vi "CPP_Aeroprobe_TimeSeries-AeroFlow.vi"() -> (5 "Plug in titles":string[](array[string]), 7 "Plug in values":string[](array[string]))   [LabVIEW 2021]
uses:
  Globals/Meas_global.vi
panel:
  in  "Downsampler":i32=10
  in  "Graphs":bool=TRUE
  out "AvgReduction (ms)":dbl
  out "reduction ms":u32
  in  "Correction File Path":path=path "M:/Preferences/Rig_Setups/All_Rigs/TubingCompensation/5HPTubingCorrection12066.xls"
  in  "Apply Phase Correction?":bool=TRUE
  out "DataArray":dbl[](array[numeric])
  out "Zeroes":dbl[](array[numeric])
  # "!! 5-hole 1-5 must be connected to Channels 1-5 !!"
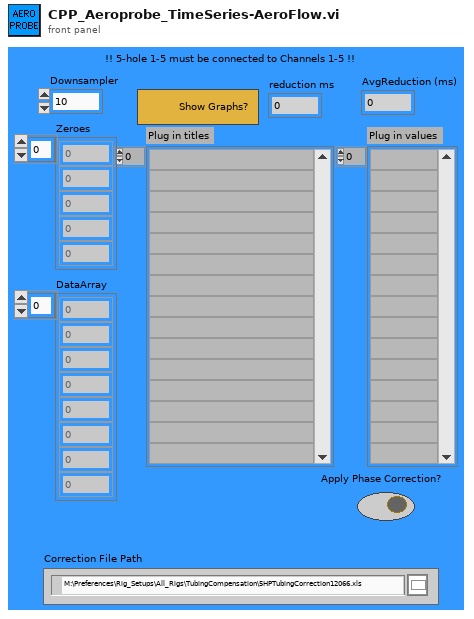
[diagram p1: front panel]
types:
  T1 = typedef "Analysis_info_cluster.ctl" = cluster{"Colour":u32, "Inst type":T2, "Inst name":string, "Symbol":string, "Code name":string, "Extra Info":string, "Inst Array":T3, "Extra Titles":string[], "Extra Values":string[], "U":dbl, "u^2":dbl, "u^3":dbl, "u^4":dbl, "Skew_u":dbl, "Kurt_u":dbl, "Sd Error in Mean":dbl, "% u'/U":dbl, "X":dbl, "Y":dbl, "Z":dbl, "Timescale integral to 25%":dbl, "Sd Error in Variance":dbl, "Calib File":path, "Calib Constants":dbl[], "Output Position":bool, "Full Stats":bool, "Av Sampling Rate":dbl, "Av No of Samples":dbl, "Total Meas Time (s)":dbl, "ADAM Ch Name":string}
  T2 = typedef "Inst_type.ctl" = enum16{"Propeller anemometer", "Raw voltage", "Pressure Transducer", "Pitot-static tube", "Preston tube", "Hot wire", "Cross wire 1", "Cross wire 2", "Generic Linear", "Generic Polynomial", "Generic BackPoly", "Fast FID", "Thermocouple", "Cold wire", "Pulsed Wire", "LDA Vel", "LDA Tran time", "LDA Arr time"}
  T3 = typedef "Instrument_Array.ctl" = enum16{"PWA", "LDA", "Analogue"}
  T4 = cluster{"Analysis Info cluster[0]":T1, "Analysis Info cluster[1]":T1, "Analysis Info cluster[2]":T1, "Analysis Info cluster[3]":T1, "Analysis Info cluster[4]":T1, "Analysis Info cluster[5]":T1, "Analysis Info cluster[6]":T1}
  T5 = typedef "Time_Trace_Cluster.ctl" = cluster{"Weighting":dbl[], "Time (s)":dbl[], "Voltage":dbl[], "Eng Values":dbl[]}
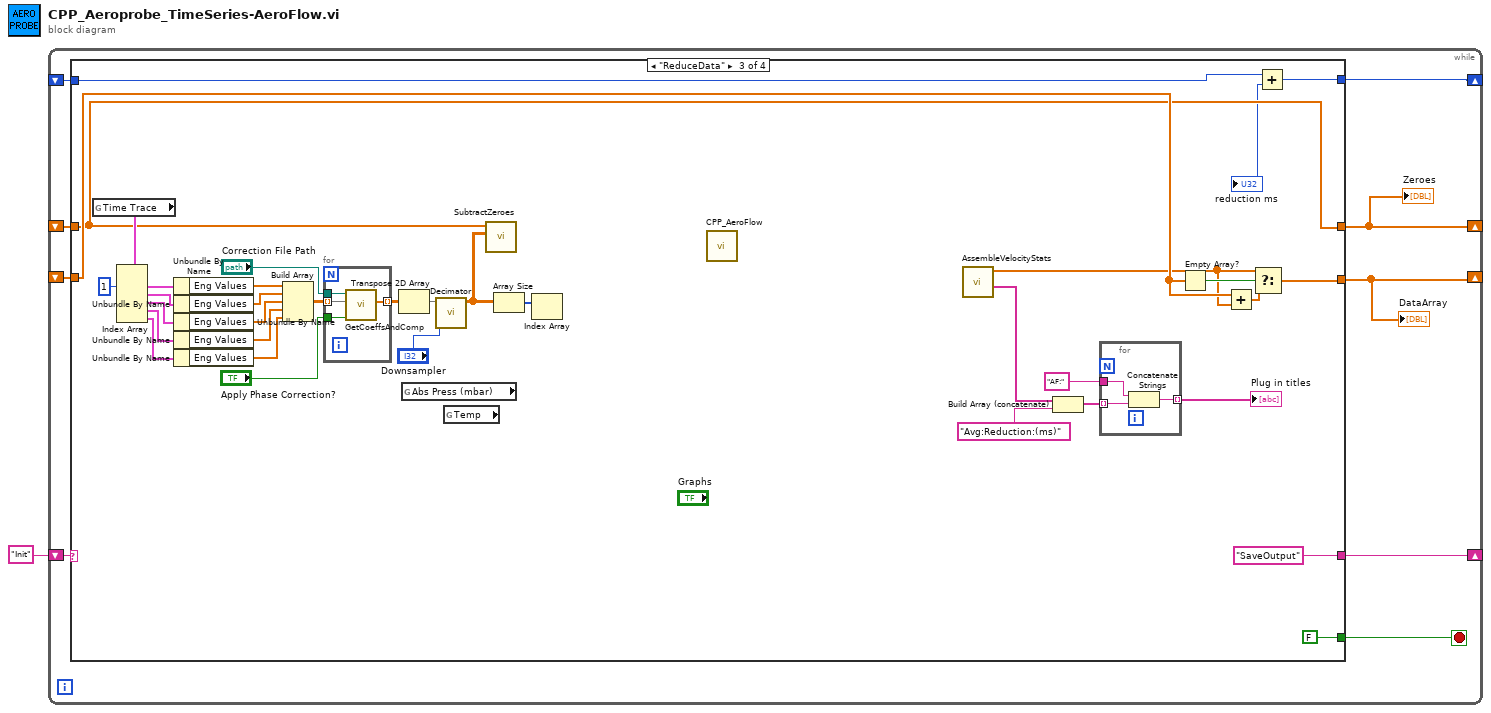
[diagram p0: block diagram]
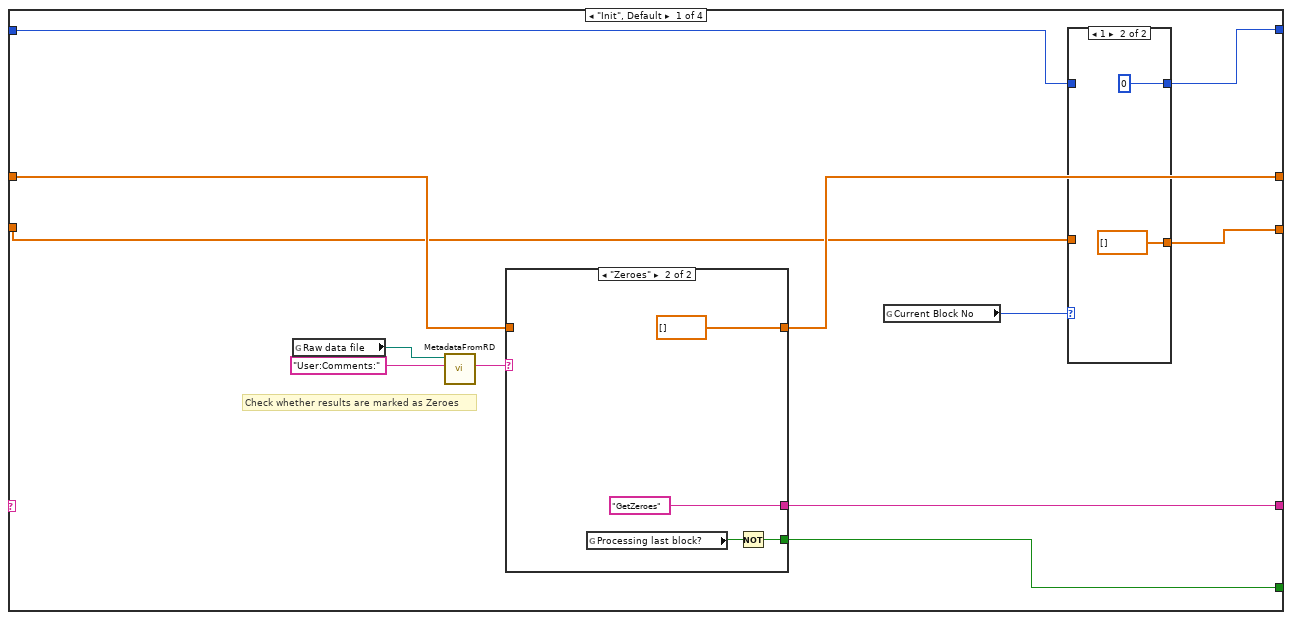
[diagram p2: hidden frame]
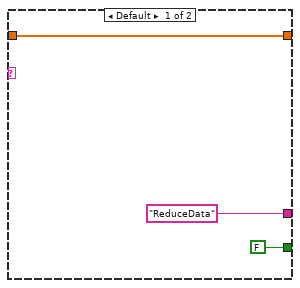
[diagram p4: hidden frame]
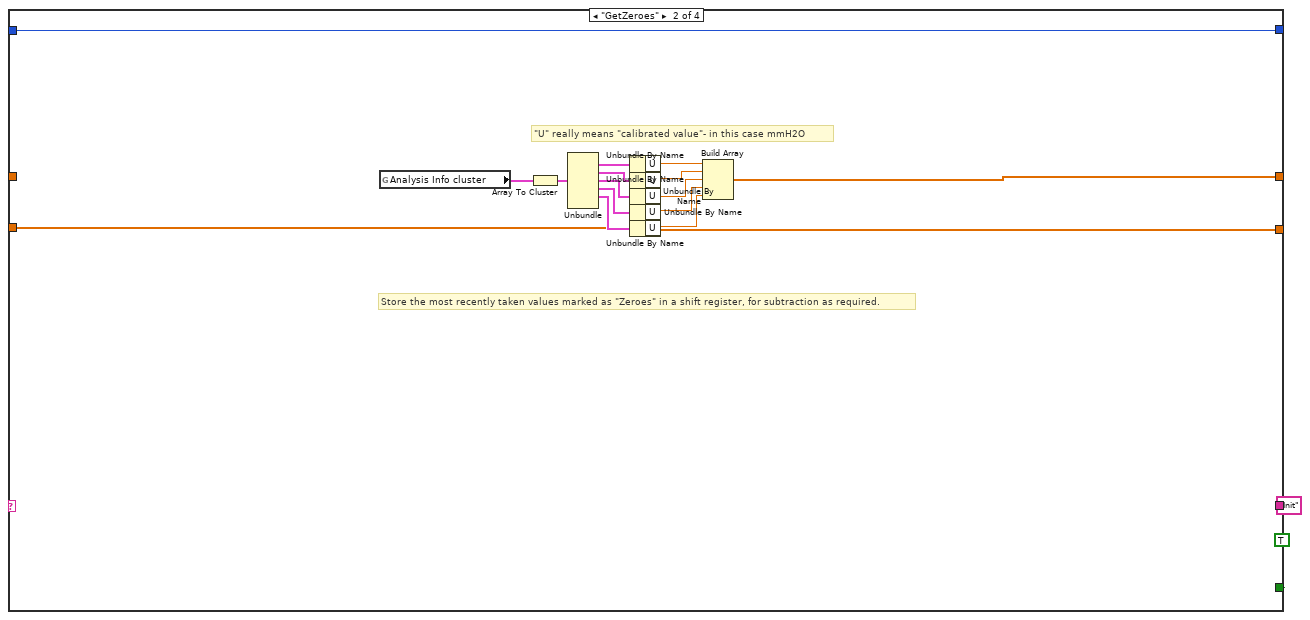
[diagram p5: hidden frame]
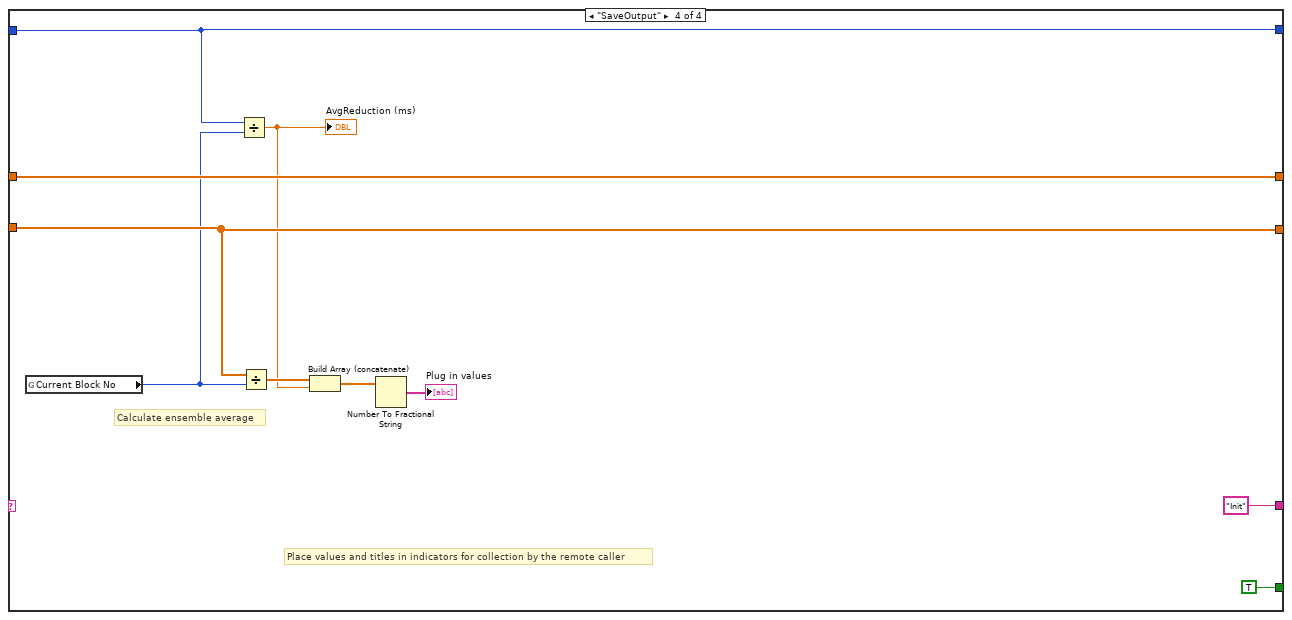
[diagram p6: hidden frame]
diagram:
  n1 = while {
    shift-right: [w9] -> _
    shift-left: "Init" -> [w10]
    shift-right: [w8] -> _
    shift-left: _ -> [w7]
    shift-right: [w6] -> _
    shift-left: _ -> [w5]
    shift-right: [w3] -> _
    shift-left: _ -> [w2]
    stop <- w4 stop-if-true
    n2 = case shown="\"ReduceData\"" w10 {
      tunnel: [w22 "Init" "SaveOutput" "Init"] -> w9
      tunnel: [w16 w37 w69 w108] -> w8
      tunnel: w7 -> [w17 _ w69 w108]
      tunnel: [w14 w35 w76 w104] -> w6
      tunnel: w5 -> [w13 w35 w77 w104]
      tunnel: [w18 TRUE FALSE TRUE] -> w4
      tunnel: [w12 w34 w63 w103] -> w3
      tunnel: w2 -> [w11 w34 w62 w103]
      frame "Init", Default {
        # "Check whether results are marked as Zeroes"
        n3 = global read "Meas_global.vi" "Raw data file"() -> (w21:path)
        n4 = call "MetadataFromRD.vi"("ChannelName"="User:Comments:", "Raw data file"=w21) -> ("ValueString"=w19:string)  [unwired: 8 in, 1 out]
        n5 = case shown="\"Zeroes\"" w19 {
          tunnel: ["ReduceData" "GetZeroes"] -> w22
          tunnel: [FALSE w32] -> w18
          tunnel: w17 -> [w27 _]
          tunnel: [w27 dbl[] [] ("t")] -> w16
          frame Default {
          }
          frame "Zeroes" {
            n6 = global read "Meas_global.vi" "Processing last block?"() -> (w31:bool)
            n7 = Not(x=w31) -> (.not. x?=w32:bool)
          }
        }
        n8 = global read "Meas_global.vi" "Current Block No"() -> (w15:i32)
        n9 = case shown="1" w15 {
          tunnel: [w24 dbl[] [] ("t")] -> w14
          tunnel: w13 -> [w24 _]
          tunnel: [w23 u32 0] -> w12
          tunnel: w11 -> [w23 _]
          frame 0, Default {
          }
          frame 1 {
          }
        }
      }
      frame "GetZeroes" {
        # "Store the most recently taken values marked as \"Zeroes\" in a shift register, for subtraction as required."
        # "\"U\" really means \"calibrated value\"- in this case mmH2O"
        n10 = global read "Meas_global.vi" "Analysis Info cluster"() -> (w39:T1[])
        n11 = Array To Cluster(array=w39) -> (cluster=w45:T4)
        n12 = Unbundle(w45) -> ("Analysis Info cluster[1]"=w46:T1, "Analysis Info cluster[2]"=w47:T1, "Analysis Info cluster[3]"=w48:T1, "Analysis Info cluster[4]"=w49:T1, "Analysis Info cluster[5]"=w50:T1)  [unwired: 2 out]
        n13 = Unbundle By Name(w46) -> ("U"=w44:dbl)
        n14 = Unbundle By Name(w47) -> ("U"=w43:dbl)
        n15 = Unbundle By Name(w48) -> ("U"=w42:dbl)
        n16 = Unbundle By Name(w49) -> ("U"=w41:dbl)
        n17 = Unbundle By Name(w50) -> ("U"=w40:dbl)
        n18 = Build Array(w44, w43, w42, w41, w40) -> (w37:dbl[])
      }
      frame "ReduceData" {
        n19 = global read "Meas_global.vi" "Time Trace"() -> (w81:T5[])
        n20 = Index Array(array=w81, index #1=1 ("index")) -> (element #1=w80:T5, element #2=w89:T5, element #3=w88:T5, element #4=w87:T5, element #5=w86:T5)  [unwired: 4 in]
        n21 = Unbundle By Name(w80) -> ("Eng Values"=w79:dbl[])
        n22 = Unbundle By Name(w89) -> ("Eng Values"=w85:dbl[])
        n23 = Unbundle By Name(w88) -> ("Eng Values"=w84:dbl[])
        n24 = Unbundle By Name(w87) -> ("Eng Values"=w83:dbl[])
        n25 = Unbundle By Name(w86) -> ("Eng Values"=w82:dbl[])
        n26 = Build Array(w79, w85, w84, w83, w82) -> (w75:dbl[][])
        n27 = for {
          tunnel: w75 -> [w98] mode=indexing
          tunnel: [w97] -> w72 mode=indexing
          tunnel: "Apply Phase Correction?" -> [w96]
          tunnel: "Correction File Path" -> [w95]
          n28 = call "GetCoeffsAndComp.vi"("Apply Phase Correction?"=w96, "mutedData"=w98, "TubingCorrectionFile"=w95) -> ("boostedData"=w97:dbl[])  [unwired: 8 in]
        }
        n29 = Transpose 2D Array(2D array=w72) -> (transposed array=w65:dbl[][])
        n30 = global read "Meas_global.vi" "Abs Press (mbar)"() -> (w71:dbl)
        n31 = call "Decimator.vi"("Decimator"="Downsampler", "Array In"=w65) -> ("DecimatedArrayOut"=w64:dbl[][])  [unwired: 9 in]
        n32 = global read "Meas_global.vi" "Temp"() -> (w67:dbl)
        n33 = call "SubtractZeroes.vi"("RawPressure"=w64, "Zeroes"=w69) -> ("ZeroedPressure"=w70:dbl[][])  [unwired: 9 in]
        n34 = Array Size(array=w64) -> (size(s)=w68:i32[])
        n35 = Index Array(array=w68) -> ()  [unwired: 1 in, 1 out]
        n36 = call "CPP_AeroFlow.vi"() -> ()  [unwired: 6 in, 4 out]
        n37 = call "AssembleVelocityStats.vi"() -> ("Plug in titles"=w52:string[], "StatsArray"=w58:dbl[], "TitlePrefix"=w54:string, 11:w55)  [unwired: 8 in]
        n38 = Build Array (concatenate)(w52, "Avg:Reduction:(ms)") -> (w53:string[])
        n39 = for {
          tunnel: w53 -> [w94] mode=indexing
          tunnel: "AF:" -> [w93]
          tunnel: [w92] -> w56 mode=indexing
          n40 = Concatenate Strings(w93, w94) -> (w92:string)
        }
        "Plug in titles" <- w56
        n41 = Empty Array?(array=w77) -> (empty?=w60:bool)
        n42 = Add(x=w77, y=w58) -> (x+y=w59:dbl[])
        n43 = Select(t=w58, s=w60, f=w59) -> (s? t:f=w76:dbl[])
        n44 = Add(x=w62) -> (y=→"reduction ms":u32, x+y=w63:u32)
      }
      frame "SaveOutput" {
        # "Place values and titles in indicators for collection by the remote caller"
        # "Calculate ensemble average"
        n45 = global read "Meas_global.vi" "Current Block No"() -> (w99:i32)
        n46 = Divide(x=w103, y=w99) -> (x/y=w100:dbl)
        "AvgReduction (ms)" <- w100
        n47 = Divide(x=w104, y=w99) -> (x/y=w102:dbl[])
        n48 = Build Array (concatenate)(w102, w100) -> (w101:dbl[])
        n49 = Number To Fractional String(number=w101) -> (F-format string=→"Plug in values":string[])  [unwired: 3 in]
      }
    }
    "Zeroes" <- w8
    "DataArray" <- w6
  }
